vi "Plotting.vi"(0 "Display Fast Loop":bool, 5 "Display Slow Loop":bool, 7 "Fast Loop State in":T3, 9 "Slow Loop State in":T1 {"Phi Setpoint" format="%#_13g"}, 11 "error in (no error)":errorcluster) -> (4 "U plot":cluster{"U saturated":sgl, "U":dbl}, 8 "Theta (Deg)":dbl, 10 "Theta Ref Plot":T2, 15 "error out":errorcluster)   [LabVIEW 2014]
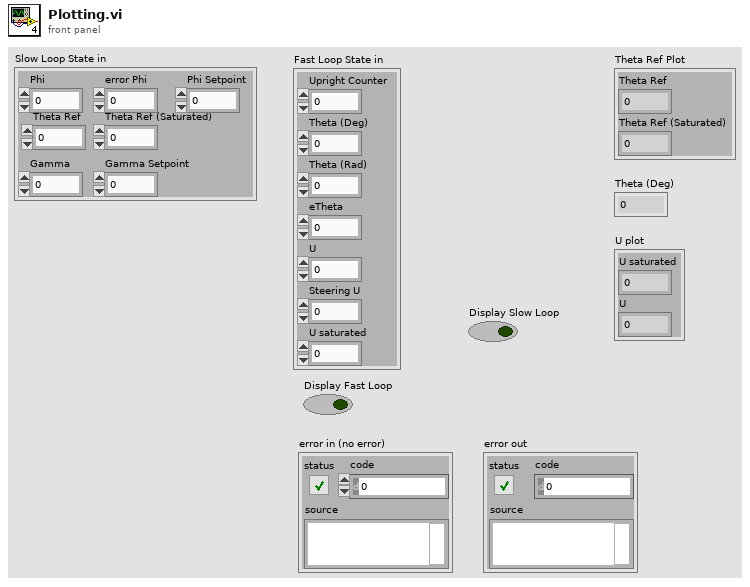
[diagram p1: front panel]
types:
  T1 = cluster{"Phi":dbl, "error Phi":dbl, "Gamma":dbl, "Theta Ref":dbl, "Theta Ref (Saturated)":sgl, "Gamma Setpoint":dbl, "Phi Setpoint":dbl}
  T2 = cluster{"Theta Ref":dbl, "Theta Ref (Saturated)":sgl}
  T3 = cluster{"Upright Counter":dbl, "Theta (Deg)":dbl, "Theta (Rad)":dbl, "eTheta":dbl, "U":dbl, "Steering U":dbl, "U saturated":sgl}
  T4 = cluster{"Theta Ref (Saturated)":sgl, "Theta Ref":dbl}
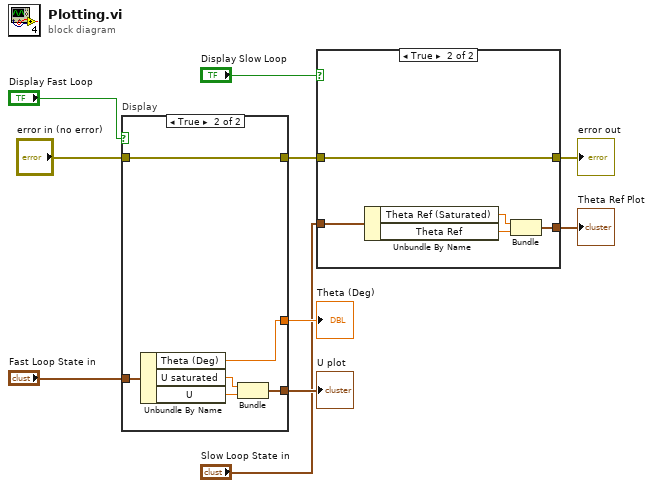
[diagram p0: block diagram]
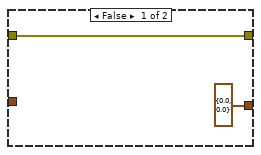
[diagram p2: hidden frame]
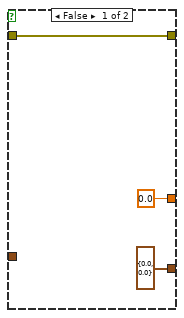
[diagram p3: hidden frame]
diagram:
  n1 = case "Display" shown="True" "Display Fast Loop" {
    tunnel: "error in (no error)" -> [w13 w17]
    tunnel: [w13 w17] -> w5
    tunnel: [cluster{"U saturated":sgl, "U":dbl} {"U saturated"=0.0, "U"=0.0} w16] -> w7
    tunnel: "Fast Loop State in" -> [_ w15]
    tunnel: [0.0 ("Theta (Deg)") w14] -> w10
    frame False {
    }
    frame True {
      n2 = Unbundle By Name(w15) -> ("Theta (Deg)"=w14:dbl, "U saturated"=w19:sgl, "U"=w18:dbl)
      n3 = Bundle("U saturated"=w19, "U"=w18) -> (w16:cluster{"U saturated":sgl, "U":dbl})  [unwired: 1 in]
    }
  }
  "Theta (Deg)" <- w10
  "U plot" <- w7
  n4 = case shown="True" "Display Slow Loop" {
    tunnel: w5 -> [w21 w26]
    tunnel: [w21 w26] -> w6
    tunnel: [T2 {"Theta Ref"=0.0, "Theta Ref (Saturated)"=0.0} w25] -> w8
    tunnel: "Slow Loop State in" -> [_ w24]
    frame False {
    }
    frame True {
      n5 = Unbundle By Name(w24) -> ("Theta Ref (Saturated)"=w23:sgl, "Theta Ref"=w22:dbl)
      n6 = Bundle("Theta Ref (Saturated)"=w23, "Theta Ref"=w22) -> (w25:T4)  [unwired: 1 in]
    }
  }
  "Theta Ref Plot" <- w8
  "error out" <- w6
